vi "Log Alarm.vi"(8 "error in (no error)":errorcluster, 10 "Message":string, 11 "Actor API":refnum<class "Alarms Handler Actor API.lvclass">) -> (0 "error out":errorcluster)   [LabVIEW 2020, in "Alarms Handler Actor API.lvclass"]
uses:
  Alarms Handler Actor API.lvclass
  C:/dev/PGS/2001 - TBCM/Source/RT/RTAF/Source/RTAF/Actors/Base Actor/API/Actor API.lvclass
  Base Actor/API/Actor API.lvclass/Actor API.ctl
  Base Actor/API/Actor API.lvclass
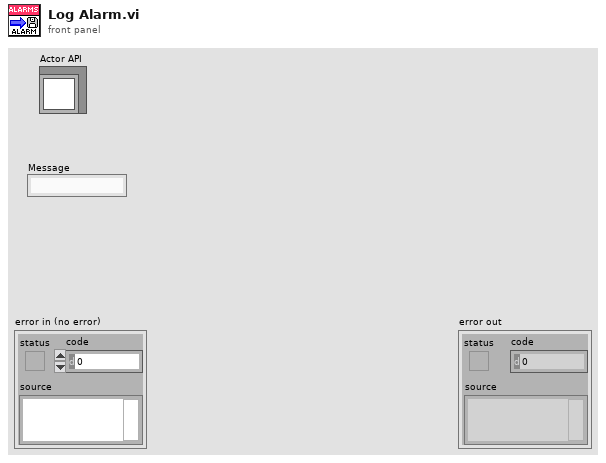
[diagram p1: front panel]
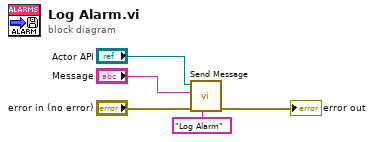
[diagram p0: block diagram]
diagram:
  n1 = call "Send Message.vi"("Name"="Log Alarm", "error in (no error)"="error in (no error)", "Payload"="Message", "Actor API in"="Actor API") -> ("error out"=→"error out":errorcluster)  [unwired: 7 in]
